vi "API - On Demand - Read 1 Analog Input Sample on Demand.vi"(8 "error in":errorcluster, 10 "Analog Input Channel Number":i32, 11 "DAQiFi Device Properties In":T1) -> (0 "error out":errorcluster, 2 "Analog Input Data Out":dbl, 3 "DAQiFi Device Properties Out":T1)   [LabVIEW 2021]
doc: "Read a single ADC measurement from the DAQ.\n-Enable channel\n-Start streaming of data\n-Download 1 datapoint\n-Stop streaming of data"
uses:
  TypeDefs/TypeDef - Cluster of DAQiFi Device Properties.ctl
  TypeDefs/Enum - Connection Type.ctl
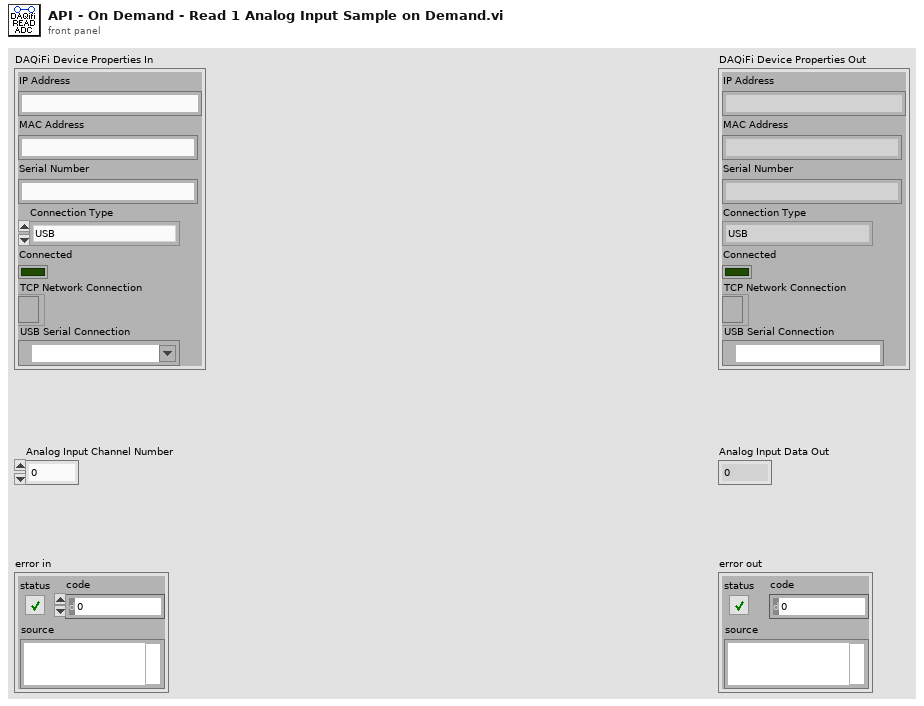
[diagram p1: front panel]
types:
  T1 = typedef "TypeDef - Cluster of DAQiFi Device Properties.ctl" = cluster{"IP Address":string, "MAC Address":string, "Serial Number":string, "Connection Type":T2, "Connected":bool, "TCP Network Connection":refnum<k5>, "USB Serial Connection":refnum<visa-resource-name>}
  T2 = typedef "Enum - Connection Type.ctl" = enum16{"USB", "TCP"}
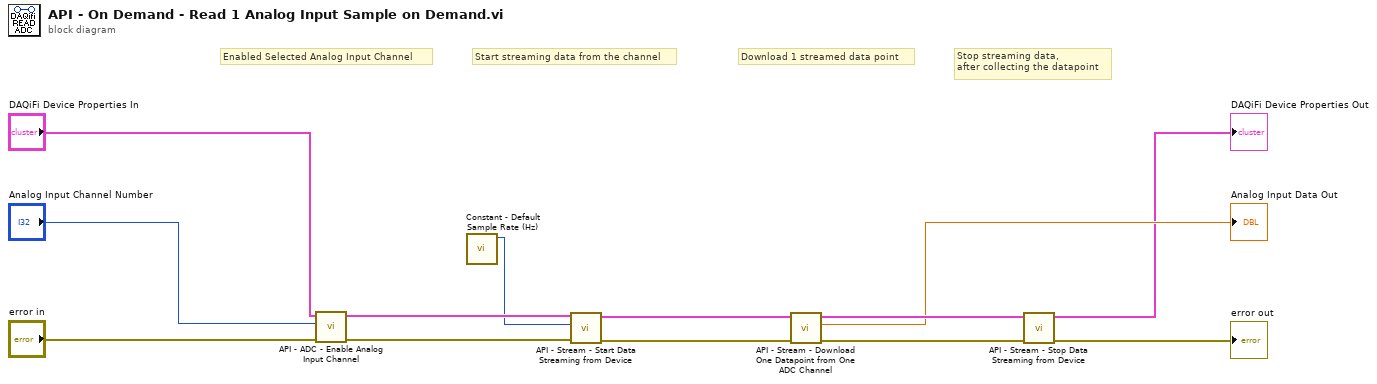
[diagram p0: block diagram]
diagram:
  # "Download 1 streamed data point"
  # "Enabled Selected Analog Input Channel"
  # "Stop streaming data,\nafter collecting the datapoint"
  # "Start streaming data from the channel"
  n1 = call "API - ADC - Enable Analog Input Channel.vi"("error in (no error)"="error in", "Analog Input Channel Number"="Analog Input Channel Number", "DAQiFi Device Properties In"="DAQiFi Device Properties In") -> ("error out"=w4:errorcluster, "DAQiFi Device Properties Out"=w5:T1)  [unwired: 7 in]
  n2 = call "Constant - Default Sample Rate (Hz).vi"() -> ("Streaming Rate (Hz)"=w3:i32)  [unwired: 11 in]
  n3 = call "API - Stream - Start Data Streaming from Device.vi"("error in"=w4, "Streaming Rate (Hz)"=w3, "DAQiFi Device Properties In"=w5) -> ("error out"=w9:errorcluster, "DAQiFi Device Properties Out"=w10:T1)  [unwired: 7 in]
  n4 = call "API - Stream - Download One Datapoint from One ADC Channel.vi"("error in"=w9, "DAQiFi Device Properties In"=w10) -> ("error out"=w12:errorcluster, "Analog Voltage (V)"=→"Analog Input Data Out":dbl, "DAQiFi Device Properties Out"=w13:T1)  [unwired: 7 in]
  n5 = call "API - Stream - Stop Data Streaming from Device.vi"("error in"=w12, "DAQiFi Device Properties In"=w13) -> ("error out"=→"error out":errorcluster, "DAQiFi Device Properties Out"=→"DAQiFi Device Properties Out":T1)  [unwired: 8 in]
